vi "worksheet embed image.vi"(7 "filename":string, 8 "error in (no error)":errorcluster, 9 "col":u16, 10 "row":u32, 11 "worksheet":u32) -> (0 "error out":errorcluster, 3 "function return":u32(ring))   [LabVIEW 8.6]
doc: "lxw_error worksheet_embed_image(lxw_worksheet worksheet, lxw_row_t row, lxw_col_t col, const char *filename);"
uses:
  pending_lvxlsxwriter/xlsxwriter.dll
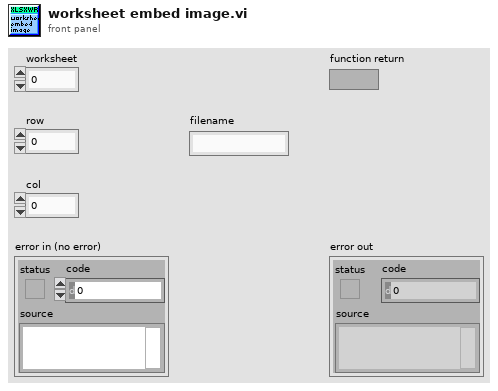
[diagram p1: front panel]
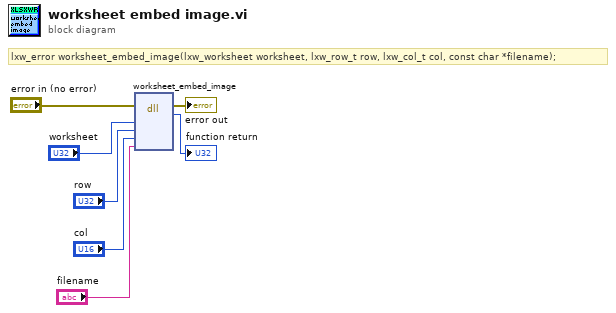
[diagram p0: block diagram]
diagram:
  # "lxw_error worksheet_embed_image(lxw_worksheet worksheet, lxw_row_t row, lxw_col_t col, const char *filename);"
  n1 = dll-call lib="C:/Users/WDAGUtilityAccount/Desktop/pending_lvxlsxwriter/xlsxwriter.*" fn="worksheet_embed_image"(error in="error in (no error)", "worksheet"="worksheet", "row"="row", "col"="col", "filename"="filename") -> (error out=→"error out":errorcluster, →"function return":u32)  [unwired: 6 in, 1 out]
